vi "subImage_UpdateLocIndicator.vi"(4 "Camera View Indicator Ref":refnum<vi>, 6 "Image Refnum":refnum<vi>, 7 "ROI":T1={"Bin"=2, "ROI"={"x offset"=256, "y offset"=256, "x width"=512, "y width"=512}} {"ROI"."x offset" min=1 max=512 step=1; "ROI"."y offset" min=1 max=512 step=1; "ROI"."x width" min=1 max=512 step=1; "ROI"."y width" min=1 max=512 step=1; "Bin" items=["1x1"=1, "2x2"=2, "4x4"=4]}, 8 "error in":errorcluster, 11 "Handle in":u32) -> (0 "error out":errorcluster, 3 "Handle out":u32)   [LabVIEW 2015]
panel:
  out "Image Graph scale":T2={"X min"=0, "Y min"=0, "X max"=2048, "Y max"=2048} {"X min" min=1 max=512 step=1; "Y min" min=1 max=512 step=1; "X max" min=1 max=512 step=1; "Y max" min=1 max=512 step=1}
  # "This sub-VI takes in ROI information and plot it onto the location indicator, and set the graph scale"
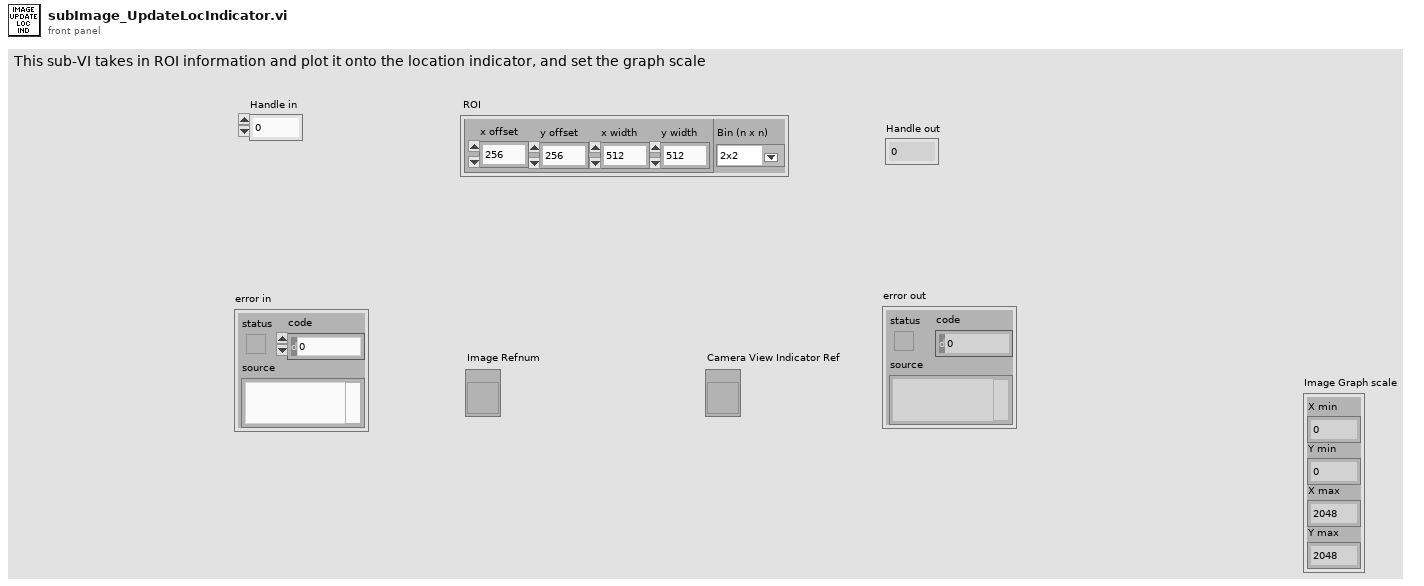
[diagram p1: front panel]
types:
  T1 = cluster{"Bin":u16, "ROI":cluster{"x offset":i32, "y offset":i32, "x width":i32, "y width":i32}}
  T2 = cluster{"X min":i32, "Y min":i32, "X max":i32, "Y max":i32}
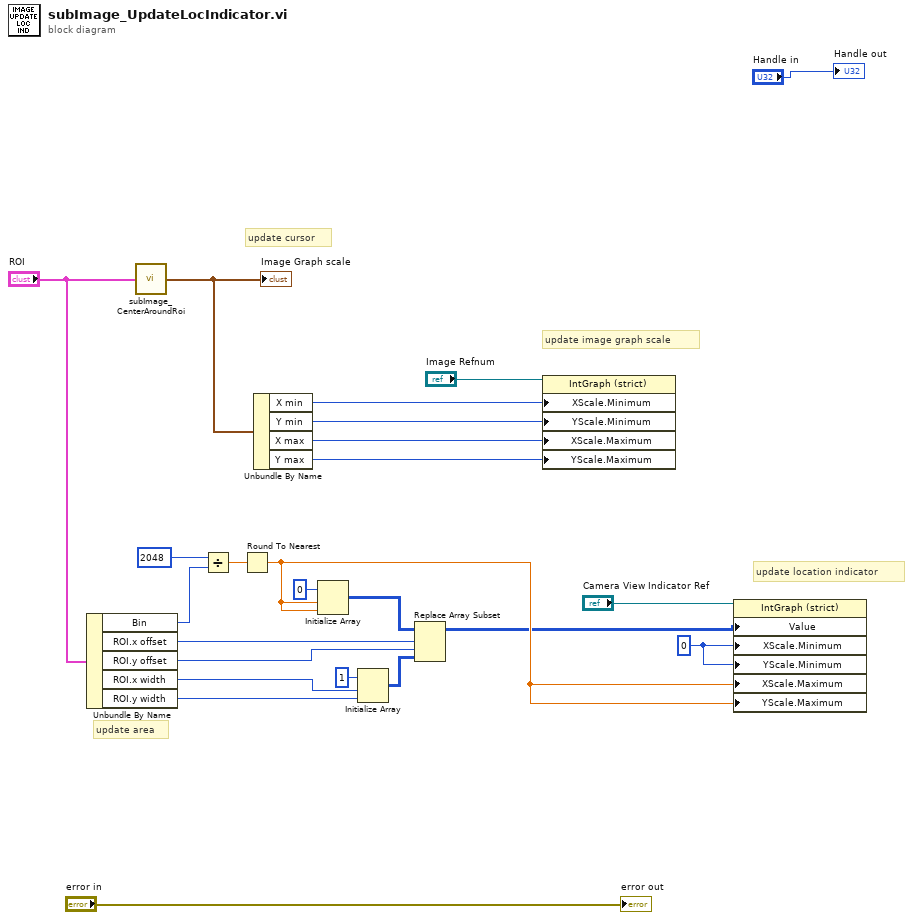
[diagram p0: block diagram]
diagram:
  w5 = 0 ("X Scale.Range:Minimum")
  # "update image graph scale"
  # "update area"
  # "update cursor"
  # "update location indicator"
  n1 = Unbundle By Name("ROI") -> ("Bin"=w17:u16, "ROI.x offset"=w16:i32, "ROI.y offset"=w15:i32, "ROI.x width"=w14:i32, "ROI.y width"=w13:i32)
  n2 = call "subImage_CenterAroundRoi.vi"("ROI in"="ROI") -> ("Graph scale"=w20:T2)
  "Image Graph scale" <- w20
  n3 = Divide(x=2048 ("Binned pixels"), y=w17) -> (x/y=w19:dbl)
  n4 = Round To Nearest(number=w19) -> (nearest integer value=w4:dbl)
  n5 = Unbundle By Name(w20) -> ("X min"=w9:i32, "Y min"=w8:i32, "X max"=w7:i32, "Y max"=w6:i32)
  n6 = Initialize Array(u16 0 ("element"), w4, w4) -> (w22:u16[][])
  n7 = Initialize Array(u16 1 ("element"), w14, w13) -> (w21:u16[][])
  n8 = Replace Array Subset(array=w22, new element=w21, index (row)=w16, index (col)=w15) -> (w3:u16[][])
  n9 = property class="IntGraph (strict)"(reference="Image Refnum", "XScale.Minimum"=w9, "YScale.Minimum"=w8, "XScale.Maximum"=w7, "YScale.Maximum"=w6) -> ()  [unwired: 1 in, 2 out]
  n10 = property class="IntGraph (strict)"(reference="Camera View Indicator Ref", "Value"=w3, "XScale.Minimum"=w5, "YScale.Minimum"=w5, "XScale.Maximum"=w4, "YScale.Maximum"=w4) -> ()  [unwired: 1 in, 2 out]
  "error out" <- "error in"
  "Handle out" <- "Handle in"
